vi "run_shutdown_splash.vi"(8 "error in (no error)":errorcluster, 11 "VI in":refnum<vi>) -> ()   [LabVIEW 2015]
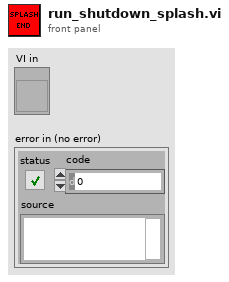
[diagram p1: front panel]
types:
  T1 = enum32{"Invalid", "Standard", "Closed", "Hidden", "Minimized", "Maximized"}
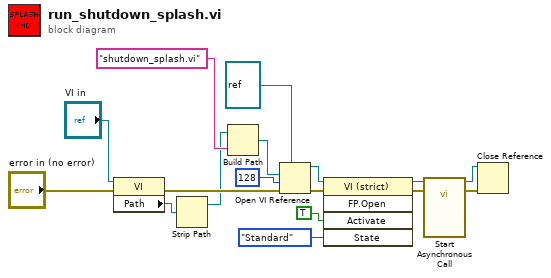
[diagram p0: block diagram]
diagram:
  n1 = property class="VI"(reference="VI in", error in="error in (no error)") -> (error out=w17:errorcluster, "Path"=w9:path)  [unwired: 1 out]
  n2 = Strip Path(path=w9) -> (stripped path=w10:path)  [unwired: 1 out]
  n3 = Build Path(base path=w10, name or relative path="shutdown_splash.vi") -> (appended path=w12:path)
  n4 = Open VI Reference(type specifier VI Refnum (for type only)=refnum<vi> refnum, vi path=w12, options=128, error in (no error)=w17) -> (vi reference=w6:refnum<vi>, error out=w4:errorcluster)  [unwired: 2 in]
  n5 = invoke class="VI (strict)" method="FP.Open"(reference=w6, error in=w4, "Activate"=TRUE ("Activate?"), "State"=T1."Standard") -> (reference out=w5:refnum<vi>, error out=w3:errorcluster)  [unwired: 1 in, 3 out]
  n6 = call-by-ref "Start Asynchronous Call"(reference=w5, error in=w3) -> (reference out=w15:refnum<vi>, error out=w16:errorcluster)  [unwired: 12 in]
  n7 = Close Reference(reference=w15, error in (no error)=w16) -> ()  [unwired: 1 out]
